vi "EF_AnalysisThread.vi"(11 "EF_AllQRefs":T1) -> ()   [LabVIEW 2017]
uses:
  Types/EF_AllQRefs.ctl
  Types/EF_GUIThread_QRef.ctl
  Types/EF_GUIThread_QData.ctl
  Types/EF_GUIThread_QCmds.ctl
  Types/EF_DAQThread_QRef.ctl
  Types/EF_DAQThread_QData.ctl
  Types/EF_DAQThread_QCmds.ctl
  Types/EF_DataProcThread_QRef.ctl
  Types/EF_DataProcThread_QData.ctl
  Types/EF_DataProcThread_QCmds.ctl
  Types/EF_AnalysisThread_QRef.ctl
  Types/EF_AnalysisThread_QData.ctl
  Types/EF_AnalysisThread_QCmds.ctl
  Types/EF_AnalysisThread_Data.ctl
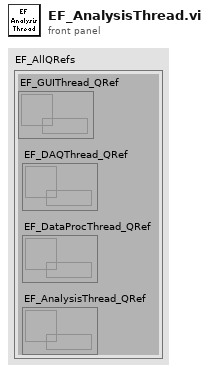
[diagram p1: front panel]
types:
  T1 = typedef "EF_AllQRefs.ctl" = cluster{"EF_GUIThread_QRef":T2, "EF_DAQThread_QRef":T3, "EF_DataProcThread_QRef":T4, "EF_AnalysisThread_QRef":T5}
  T2 = typedef "EF_GUIThread_QRef.ctl" = refnum<queue>
  T3 = typedef "EF_DAQThread_QRef.ctl" = refnum<queue>
  T4 = typedef "EF_DataProcThread_QRef.ctl" = refnum<queue>
  T5 = typedef "EF_AnalysisThread_QRef.ctl" = refnum<queue>
  T6 = typedef "EF_AnalysisThread_Data.ctl" = cluster{"DecayT0":dbl, "AvgLTs":dbl[], "HistoRes":dbl, "TotalBinsHistStart":u64[], "TimeTraceRes":dbl, "LTThreshold":dbl, "TTLActivate":bool, "TTLDelay":dbl, "TTLWidth":dbl, "MinIntCounts":u32}
  T7 = typedef "EF_GUIThread_QCmds.ctl" = enum16{"_none_", "Res", "Histo", "TTrace", "Lifetime", "Rates", "Status", "ShortDelay", "_Error_"}
  T8 = typedef "EF_GUIThread_QData.ctl" = cluster{"Histo":u32[], "Rates":i32[], "Cmd":T7, "Res":dbl, "TimeTrace":u32[], "Bin":i32, "Status":string, "Total bin":u64, "AvgLTs":dbl[], "TotalBinsHistStart":u64[], "HistStartTimes":dbl[], "MinDelays":dbl[], "ShortDelay":bool, "Pending TTLs":i32, "error in (no error)":errorcluster, "DeltaT":dbl, "NumLTs":i32}
  T9 = typedef "EF_AnalysisThread_QData.ctl" = cluster{"Cmd":T10, "Histo":u32[], "DecayT0":dbl, "HistoRes":dbl, "TotalBinHistStart":u64, "TimeTraceRes":dbl, "Total bin":u64, "TickCount":u32, "LTThreshold":dbl, "TTLActivate":bool, "TTLDelay":dbl, "TTLWidth":dbl, "MinIntCounts":u32}
  T10 = typedef "EF_AnalysisThread_QCmds.ctl" = enum16{"Exit", "CalcAvgLT", "CalcDelay", "SetDecayT0", "SetHistoRes", "SetTimeTraceRes", "SetLTThreshold", "SetTTLActiv", "SetTTLDelay", "SetTTLWidth", "SetMinIntCounts"}
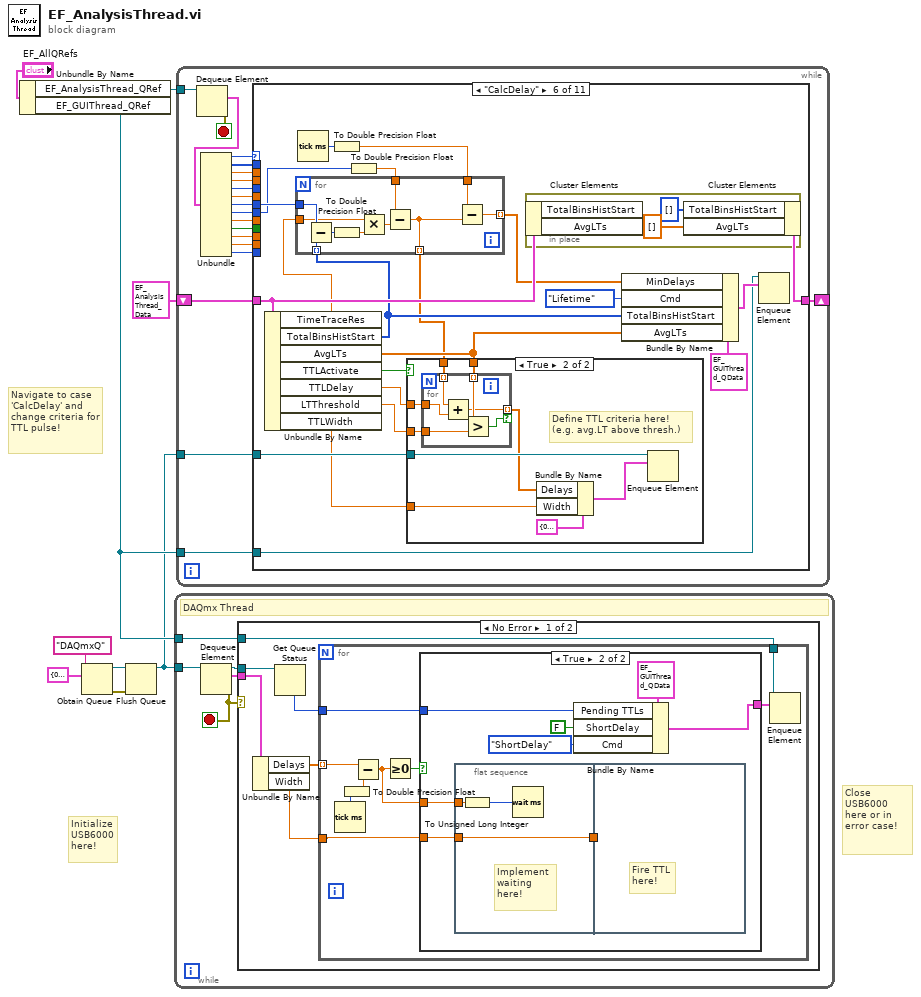
[diagram p0: block diagram]
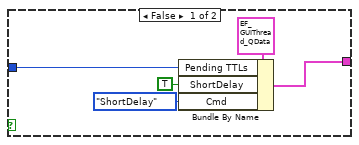
[diagram p2: hidden frame]
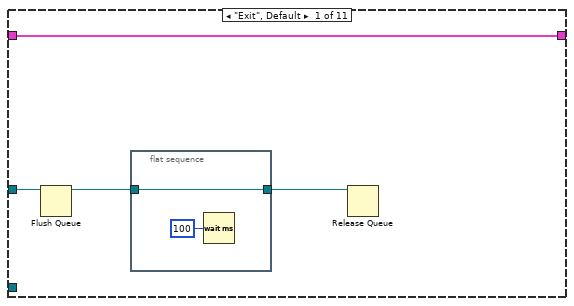
[diagram p4: hidden frame]
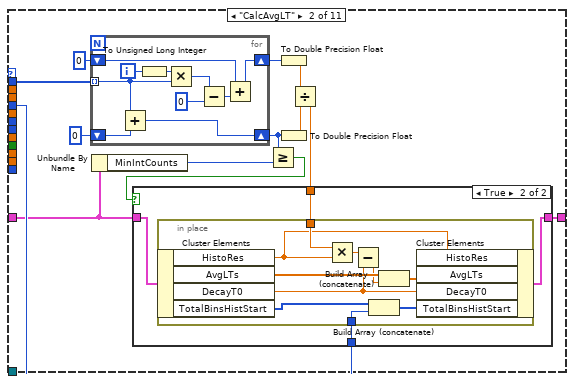
[diagram p5: hidden frame]
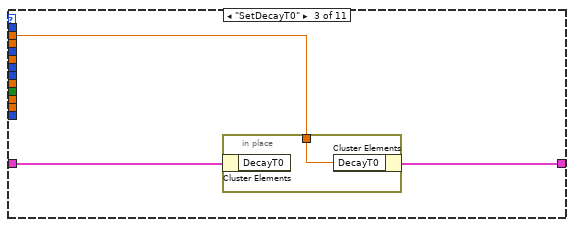
[diagram p7: hidden frame]
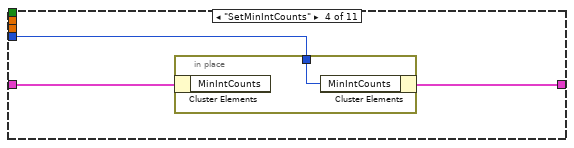
[diagram p8: hidden frame]
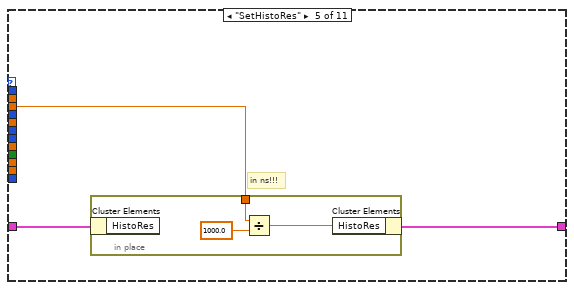
[diagram p9: hidden frame]
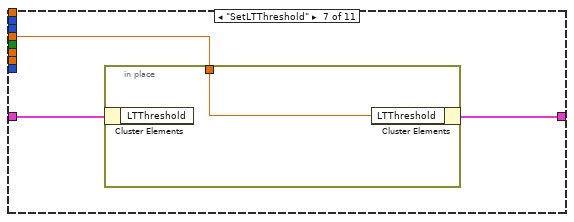
[diagram p11: hidden frame]
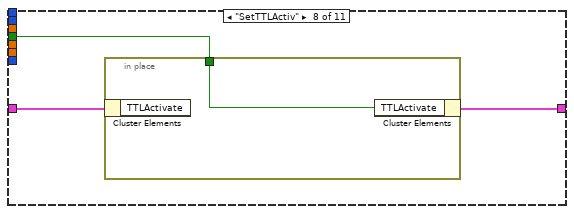
[diagram p12: hidden frame]
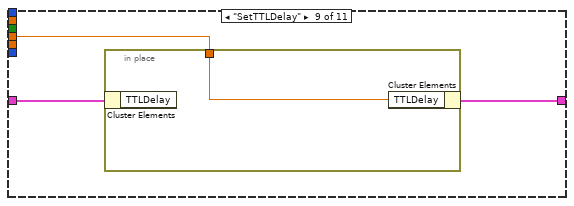
[diagram p13: hidden frame]
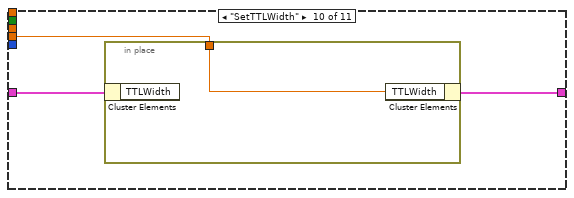
[diagram p14: hidden frame]
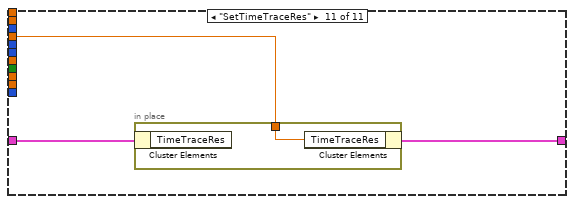
[diagram p15: hidden frame]
diagram:
  # "Navigate to case 'CalcDelay' and change criteria for TTL pulse!"
  # "Close\nUSB6000\nhere or in error case!"
  # "Initialize\nUSB6000\nhere!"
  n1 = Unbundle By Name("EF_AllQRefs") -> ("EF_AnalysisThread_QRef"=w3:T5, "EF_GUIThread_QRef"=w2:T2)
  n2 = Obtain Queue(name (unnamed)="DAQmxQ", element data type=cluster{"Width":dbl, "Delays":dbl[]} {"Width"=0.0, "Delays"=[]}) -> (queue out=w6:refnum<queue>, error out=w5:errorcluster)  [unwired: 3 in, 1 out]
  n3 = Flush Queue(queue=w6, error in (no error)=w5) -> (queue out=w1:refnum<queue>)  [unwired: 2 out]
  n4 = while {
    tunnel: w1 -> [w12]
    tunnel: w2 -> [w13]
    stop <- w11 stop-if-true
    # "DAQmx Thread"
    n5 = Dequeue Element(queue=w12) -> (queue out=w10:refnum<queue>, element=w14:cluster{"Width":dbl, "Delays":dbl[]}, error out=w11:errorcluster)  [unwired: 2 in, 1 out]
    n6 = case shown="No Error" w11 {
      tunnel: w14 -> [w17 _]
      tunnel: w13 -> [w18 _]
      tunnel: w10 -> [w16 _]
      frame No Error {
        n7 = Unbundle By Name(w17) -> ("Delays"=w20:dbl[], "Width"=w19:dbl)
        n8 = Get Queue Status(queue=w16) -> (# elements in queue=w15:i32)  [unwired: 2 in, 7 out]
        n9 = for {
          tunnel: w20 -> [w26] mode=indexing
          tunnel: w19 -> [w25]
          tunnel: w18 -> [w24]
          tunnel: w15 -> [w21]
          n10 = Tick Count (ms)() -> (millisecond timer value=w29:u32)
          n11 = To Double Precision Float(number=w29) -> (double precision float=w28:dbl)
          n12 = Subtract(x=w26, y=w28) -> (x-y=w22:dbl)
          n13 = Greater Or Equal To 0?(x=w22) -> (x >= 0?=w27:bool)
          n14 = case shown="True" w27 {
            tunnel: w22 -> [_ w42]
            tunnel: w25 -> [_ w40]
            tunnel: [w31 w36] -> w23
            tunnel: w21 -> [w30 w35]
            frame False {
              n15 = Bundle By Name(cluster=T8 {"Histo"=[], "Rates"=[], "Cmd"=enum."_none_", "Res"=0.0, "TimeTrace"=[], "Bin"=0, "Status"="", "Total bin"=0, "AvgLTs"=[], "TotalBinsHistStart"=[], "HistStartTimes"=[], "MinDelays"=[], "ShortDelay"=FALSE, "Pending TTLs"=0, "error in (no error)"={"status"=FALSE, "code"=0, "source"=""}, "DeltaT"=0.0, "NumLTs"=0} ("element"), "Pending TTLs"=w30, "ShortDelay"=TRUE, "Cmd"=EF_GUIThread_QCmds."ShortDelay") -> (w31:T8)
            }
            frame True {
              n16 = flat-sequence {
                tunnel: w42 -> [w44]
                tunnel: [w43] -> w41
                tunnel: w40 -> [w43]
                tunnel: w41 -> [_]
                frame #0 {
                  # "Implement\nwaiting\nhere!"
                  n17 = To Unsigned Long Integer(number=w44) -> (unsigned 32bit integer=w45:u32)
                  n18 = Wait (ms)(milliseconds to wait=w45) -> ()  [unwired: 1 out]
                }
                frame #1 {
                  # "Fire TTL\nhere!"
                }
              }
              n19 = Bundle By Name(cluster=T8 {"Histo"=[], "Rates"=[], "Cmd"=enum."_none_", "Res"=0.0, "TimeTrace"=[], "Bin"=0, "Status"="", "Total bin"=0, "AvgLTs"=[], "TotalBinsHistStart"=[], "HistStartTimes"=[], "MinDelays"=[], "ShortDelay"=FALSE, "Pending TTLs"=0, "error in (no error)"={"status"=FALSE, "code"=0, "source"=""}, "DeltaT"=0.0, "NumLTs"=0} ("element"), "Pending TTLs"=w35, "ShortDelay"=FALSE, "Cmd"=EF_GUIThread_QCmds."ShortDelay") -> (w36:T8)
            }
          }
          n20 = Enqueue Element(queue=w24, element=w23) -> ()  [unwired: 2 in, 3 out]
        }
      }
      frame Error {
        # "Close\nUSB6000\nhere or after loop!"
      }
    }
  }
  n21 = while {
    tunnel: w3 -> [w65]
    shift-right: [w60] -> _
    shift-left: T6 {"DecayT0"=0.0, "AvgLTs"=[], "HistoRes"=0.0, "TotalBinsHistStart"=[], "TimeTraceRes"=0.0, "LTThreshold"=0.0, "TTLActivate"=FALSE, "TTLDelay"=0.0, "TTLWidth"=0.0, "MinIntCounts"=0} ("EF_AnalysisThread_Data") -> [w59]
    tunnel: w1 -> [w48]
    tunnel: w2 -> [w47]
    stop <- w64 stop-if-true
    n22 = Dequeue Element(queue=w65) -> (element=w63:T9, error out=w64:errorcluster)  [unwired: 2 in, 2 out]
    n23 = Unbundle(w63) -> ("Cmd"=w62:T10, "Histo"=w61:u32[], "DecayT0"=w58:dbl, "HistoRes"=w57:dbl, "TotalBinHistStart"=w56:u64, "TimeTraceRes"=w55:dbl, "Total bin"=w54:u64, "TickCount"=w53:u32, "LTThreshold"=w52:dbl, "TTLActivate"=w51:bool, "TTLDelay"=w50:dbl, "TTLWidth"=w49:dbl, "MinIntCounts"=w46:u32)
    n24 = case shown="\"CalcDelay\"" w62 {
      tunnel: w61 -> [_ w83 _ _ _ _ _ _ _ _ _]
      tunnel: [w69 w78 w111 w115 w119 w144 w172 w177 w181 w185 w188] -> w60
      tunnel: w59 -> [w69 w75 w112 w116 w120 w137 w174 w178 w182 w186 w190]
      tunnel: w58 -> [_ _ w110 _ _ _ _ _ _ _ _]
      tunnel: w57 -> [_ _ _ _ w118 _ _ _ _ _ _]
      tunnel: w56 -> [_ w76 _ _ _ _ _ _ _ _ _]
      tunnel: w55 -> [_ _ _ _ _ _ _ _ _ _ w189]
      tunnel: w54 -> [_ _ _ _ _ w140 _ _ _ _ _]
      tunnel: w53 -> [_ _ _ _ _ w132 _ _ _ _ _]
      tunnel: w52 -> [_ _ _ _ _ _ w173 _ _ _ _]
      tunnel: w51 -> [_ _ _ _ _ _ _ w176 _ _ _]
      tunnel: w50 -> [_ _ _ _ _ _ _ _ w180 _ _]
      tunnel: w49 -> [_ _ _ _ _ _ _ _ _ w184 _]
      tunnel: w48 -> [w68 _ _ _ _ w135 _ _ _ _ _]
      tunnel: w47 -> [_ _ _ _ _ w124 _ _ _ _ _]
      tunnel: w46 -> [_ _ _ w114 _ _ _ _ _ _ _]
      frame "Exit", Default {
        n25 = Flush Queue(queue=w68) -> (queue out=w67:refnum<queue>)  [unwired: 1 in, 2 out]
        n26 = flat-sequence {
          tunnel: w67 -> [w71]
          tunnel: [w71] -> w66
          frame #0 {
            n27 = Wait (ms)(milliseconds to wait=u32 100) -> ()  [unwired: 1 out]
          }
        }
        n28 = Release Queue(queue=w66) -> ()  [unwired: 2 in, 3 out]
      }
      frame "CalcAvgLT" {
        n29 = for {
          tunnel: w83 -> [w102] mode=indexing
          shift-right: [w106] -> w81
          shift-left: u32 0 -> [w107]
          shift-right: [w101] -> w74
          shift-left: u32 0 -> [w100]
          i -> [w109]
          n30 = Add(x=w102, y=w100) -> (x+y=w101:u32)
          n31 = To Unsigned Long Integer(number=w109) -> (unsigned 32bit integer=w108:u32)
          n32 = Multiply(x=w108, y=w102) -> (x*y=w105:u32)
          n33 = Subtract(x=w105, y=u32 0) -> (x-y=w103:u32)
          n34 = Add(x=w107, y=w103) -> (x+y=w106:u32)
        }
        n35 = Unbundle By Name(w75) -> ("MinIntCounts"=w73:u32)
        n36 = Greater Or Equal?(x=w74, y=w73) -> (x >= y?=w72:bool)
        n37 = To Double Precision Float(number=w81) -> (double precision float=w82:dbl)
        n38 = To Double Precision Float(number=w74) -> (double precision float=w80:dbl)
        n39 = Divide(x=w82, y=w80) -> (x/y=w77:dbl)
        n40 = case shown="True" w72 {
          tunnel: [w85 w89] -> w78
          tunnel: w77 -> [_ w88]
          tunnel: w76 -> [_ w87]
          tunnel: w75 -> [w85 w86]
          frame False {
          }
          frame True {
            n41 = in-place {
              in-place-border: w88 -> [w95]
              in-place-border: w87 -> [w91]
              n42 = in-place-cluster #1(w86) -> ("HistoRes"=w93:dbl, "AvgLTs"=w99:dbl[], "DecayT0"=w96:dbl, "TotalBinsHistStart"=w92:u64[])
              n43 = Multiply(x=w95, y=w93) -> (x*y=w94:dbl)
              n44 = Subtract(x=w94, y=w96) -> (x-y=w97:dbl)
              n45 = Build Array (concatenate)(w92, w91) -> (w90:u64[])
              n46 = Build Array (concatenate)(w99, w97) -> (w98:dbl[])
              n47 = in-place-cluster #1("HistoRes"=w93, "AvgLTs"=w98, "DecayT0"=w96, "TotalBinsHistStart"=w90) -> (w89:T6)
            }
          }
        }
      }
      frame "SetDecayT0" {
        n48 = in-place {
          in-place-border: w110 -> [w113]
          n49 = in-place-cluster #2(w112) -> ()  [unwired: 1 out]
          n50 = in-place-cluster #2("DecayT0"=w113) -> (w111:T6)
        }
      }
      frame "SetMinIntCounts" {
        n51 = in-place {
          in-place-border: w114 -> [w117]
          n52 = in-place-cluster #3(w116) -> ()  [unwired: 1 out]
          n53 = in-place-cluster #3("MinIntCounts"=w117) -> (w115:T6)
        }
      }
      frame "SetHistoRes" {
        # "in ns!!!"
        n54 = in-place {
          in-place-border: w118 -> [w123]
          n55 = in-place-cluster #4(w120) -> ()  [unwired: 1 out]
          n56 = Divide(x=w123, y=1000.0) -> (x/y=w121:dbl)
          n57 = in-place-cluster #4("HistoRes"=w121) -> (w119:T6)
        }
      }
      frame "CalcDelay" {
        n58 = Unbundle By Name(w137) -> ("TimeTraceRes"=w136:dbl, "TotalBinsHistStart"=w129:u64[], "AvgLTs"=w130:dbl[], "TTLActivate"=w134:bool, "TTLDelay"=w126:dbl, "LTThreshold"=w133:dbl, "TTLWidth"=w127:dbl)
        n59 = Tick Count (ms)() -> (millisecond timer value=w138:u32)
        n60 = To Double Precision Float(number=w138) -> (double precision float=w139:dbl)
        n61 = To Double Precision Float(number=w132) -> (double precision float=w131:dbl)
        n62 = for {
          tunnel: w129 -> [w168] mode=indexing
          tunnel: w140 -> [w169]
          tunnel: w136 -> [w166]
          tunnel: w139 -> [w163]
          tunnel: [w162] -> w125 mode=indexing
          tunnel: w131 -> [w161]
          tunnel: [w160] -> w128 mode=indexing
          n63 = Subtract(x=w169, y=w168) -> (x-y=w167:u64)
          n64 = To Double Precision Float(number=w167) -> (double precision float=w165:dbl)
          n65 = Multiply(x=w166, y=w165) -> (x*y=w164:dbl)
          n66 = Subtract(x=w161, y=w164) -> (x-y=w160:dbl)
          n67 = Subtract(x=w163, y=w160) -> (x-y=w162:dbl)
        }
        n68 = case shown="True" w134 {
          tunnel: w135 -> [_ w153]
          tunnel: w130 -> [_ w152]
          tunnel: w133 -> [_ w151]
          tunnel: w128 -> [_ w150]
          tunnel: w127 -> [_ w148]
          tunnel: w126 -> [_ w147]
          frame False {
          }
          frame True {
            # "Define TTL criteria here!\n(e.g. avg.LT above thresh.)"
            n69 = for {
              tunnel: w152 -> [w158] mode=indexing
              tunnel: w151 -> [w159]
              tunnel: [w154] -> w145 mode=indexing if=w157
              tunnel: w150 -> [w156] mode=indexing
              tunnel: w147 -> [w155]
              n70 = Add(x=w156, y=w155) -> (x+y=w154:dbl)
              n71 = Greater?(x=w158, y=w159) -> (0:w157:bool)
            }
            n72 = Bundle By Name(cluster=cluster{"Width":dbl, "Delays":dbl[]} {"Width"=0.0, "Delays"=[]}, "Delays"=w145, "Width"=w148) -> (w149:cluster{"Width":dbl, "Delays":dbl[]})
            n73 = Enqueue Element(queue=w153, element=w149) -> ()  [unwired: 2 in, 3 out]
          }
        }
        n74 = in-place {
          n75 = in-place-cluster #5(w137) -> ()  [unwired: 2 out]
          n76 = in-place-cluster #5("TotalBinsHistStart"=u64[] [], "AvgLTs"=dbl[] []) -> (w144:T6)
        }
        n77 = Bundle By Name(cluster=T8 {"Histo"=[], "Rates"=[], "Cmd"=enum."_none_", "Res"=0.0, "TimeTrace"=[], "Bin"=0, "Status"="", "Total bin"=0, "AvgLTs"=[], "TotalBinsHistStart"=[], "HistStartTimes"=[], "MinDelays"=[], "ShortDelay"=FALSE, "Pending TTLs"=0, "error in (no error)"={"status"=FALSE, "code"=0, "source"=""}, "DeltaT"=0.0, "NumLTs"=0} ("element"), "MinDelays"=w125, "Cmd"=EF_GUIThread_QCmds."Lifetime", "TotalBinsHistStart"=w129, "AvgLTs"=w130) -> (w141:T8)
        n78 = Enqueue Element(queue=w124, element=w141) -> ()  [unwired: 2 in, 3 out]
      }
      frame "SetLTThreshold" {
        n79 = in-place {
          in-place-border: w173 -> [w175]
          n80 = in-place-cluster #6(w174) -> ()  [unwired: 1 out]
          n81 = in-place-cluster #6("LTThreshold"=w175) -> (w172:T6)
        }
      }
      frame "SetTTLActiv" {
        n82 = in-place {
          in-place-border: w176 -> [w179]
          n83 = in-place-cluster #7(w178) -> ()  [unwired: 1 out]
          n84 = in-place-cluster #7("TTLActivate"=w179) -> (w177:T6)
        }
      }
      frame "SetTTLDelay" {
        n85 = in-place {
          in-place-border: w180 -> [w183]
          n86 = in-place-cluster #8(w182) -> ()  [unwired: 1 out]
          n87 = in-place-cluster #8("TTLDelay"=w183) -> (w181:T6)
        }
      }
      frame "SetTTLWidth" {
        n88 = in-place {
          in-place-border: w184 -> [w187]
          n89 = in-place-cluster #9(w186) -> ()  [unwired: 1 out]
          n90 = in-place-cluster #9("TTLWidth"=w187) -> (w185:T6)
        }
      }
      frame "SetTimeTraceRes" {
        n91 = in-place {
          in-place-border: w189 -> [w191]
          n92 = in-place-cluster #10(w190) -> ()  [unwired: 1 out]
          n93 = in-place-cluster #10("TimeTraceRes"=w191) -> (w188:T6)
        }
      }
    }
  }
